vi "Image List Column--constant.vi"() -> (3 "columns":i32)   [LabVIEW 2021, in "TSC Button Editor.lvclass"]
doc: "This constant VI defines the number of visible columns for the image list.\n\n<b>Code Developed By:</b> +\nDaniel Coons +\nTechnology Service Corporation +\nwww.tsc.com/atcs"
uses:
  TSC Button Editor.lvclass
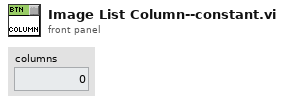
[diagram p1: front panel]
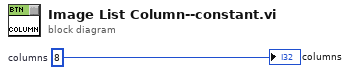
[diagram p0: block diagram]
diagram:
  w1 = 8  # columns
  "columns" <- w1
